vi "Parse Category Overrides.vi"() -> (1 "Non Localized Names":string[](array[string]), 2 "Names":string[](array[string]), 3 "Priorities":i32[](array[numeric]))   [LabVIEW 2016, in "NI_NPW_Filters.lvlib"]
uses:
  <resource>/dialog/NewProjectWizard/Filters/NI_NPW_Filters.lvlib
  <resource>/dialog/NewProjectWizard/Loading Project Info/NI_NPW_Loading Project Info.lvlib
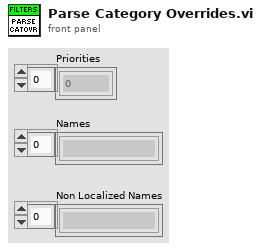
[diagram p1: front panel]
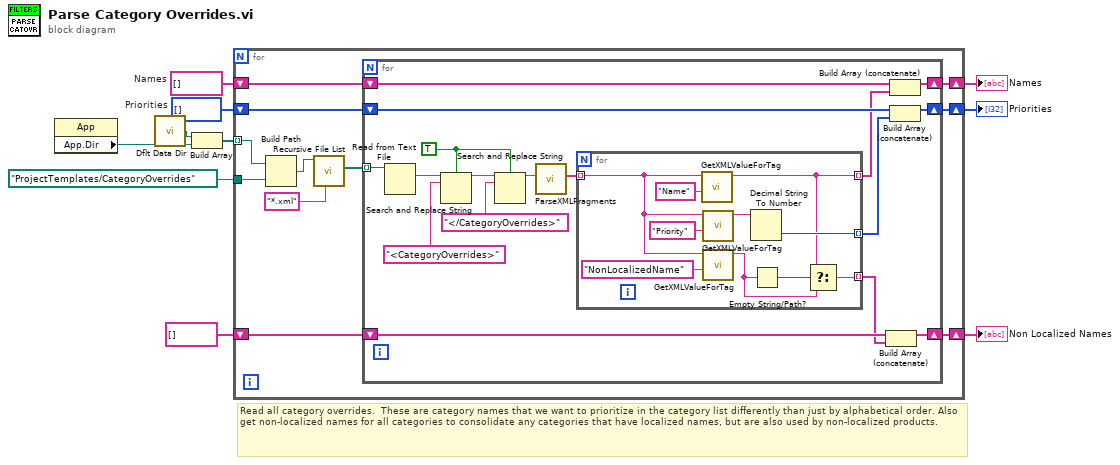
[diagram p0: block diagram]
diagram:
  w8 = i32[] []  # Priorities
  w7 = string[] []  # Names
  # "Read all category overrides.  These are category names that we want to prioritize in the category list differently than just by alphabetical order. Also get non-localized names for all categories to consolidate any categories that have localized names, but are also used by non-localized products."
  n1 = property class="App"() -> ("App.Dir"=w6:path)  [unwired: 2 in, 2 out]
  n2 = call <vilib>:"Dflt Data Dir.vi"() -> ("App:Default Data Directory"=w3:path)
  n3 = Build Array(w3, w6) -> (w4:path[])
  n4 = for {
    tunnel: w4 -> [w20] mode=indexing
    tunnel: path "ProjectTemplates/CategoryOverrides" -> [w21]
    shift-right: [w14] -> w9
    shift-left: w7 -> [w16]
    shift-right: [w13] -> w10
    shift-left: w8 -> [w15]
    shift-right: [w11] -> w1
    shift-left: string[] [] -> [w12]
    n5 = Build Path(base path=w20, name or relative path=w21) -> (appended path=w19:path)
    n6 = call <vilib>:"Recursive File List.vi"("pattern"="*.xml", "Folder Path"=w19) -> ("All Files in Dir"=w17:path[])  [unwired: 5 in, 4 out]
    n7 = for {
      tunnel: w17 -> [w38] mode=indexing
      shift-right: [w26] -> w14
      shift-left: w16 -> [w30]
      shift-right: [w25] -> w13
      shift-left: w15 -> [w29]
      shift-right: [w23] -> w11
      shift-left: w12 -> [w24]
      w34 = TRUE ("ignore case? (F)")
      n8 = Read from Text File(file (use dialog)=w38) -> (text=w36:string)  [unwired: 3 in, 3 out]
      n9 = Search and Replace String(case sensitive?=w34, input string=w36, search string="<CategoryOverrides>") -> (result string=w35:string)  [unwired: 5 in, 3 out]
      n10 = Search and Replace String(case sensitive?=w34, input string=w35, search string="</CategoryOverrides>") -> (result string=w32:string)  [unwired: 5 in, 3 out]
      n11 = call <vilib>:"ParseXMLFragments.vi"("XML in"=w32) -> ("XML Elements"=w37:string[])  [unwired: 9 in, 1 out]
      n12 = for {
        tunnel: w37 -> [w44] mode=indexing
        tunnel: [w40] -> w28 mode=indexing
        tunnel: [w45] -> w27 mode=indexing
        tunnel: [w39] -> w22 mode=indexing
        n13 = call <resource>:"GetXMLValueForTag.vi"("tag"="Name", "XML"=w44) -> ("value"=w40:string)  [unwired: 7 in, 2 out]
        n14 = call <resource>:"GetXMLValueForTag.vi"("tag"="Priority", "XML"=w44) -> ("value"=w46:string)  [unwired: 7 in, 2 out]
        n15 = call <resource>:"GetXMLValueForTag.vi"("tag"="NonLocalizedName", "XML"=w44) -> ("value"=w41:string)  [unwired: 7 in, 2 out]
        n16 = Decimal String To Number(string=w46) -> (number=w45:i32)  [unwired: 2 in, 1 out]
        n17 = Empty String/Path?(string/path=w41) -> (empty?=w42:bool)
        n18 = Select(t=w40, s=w42, f=w41) -> (s? t:f=w39:string)
      }
      n19 = Build Array (concatenate)(w24, w22) -> (w23:string[])
      n20 = Build Array (concatenate)(w30, w28) -> (w26:string[])
      n21 = Build Array (concatenate)(w29, w27) -> (w25:i32[])
    }
  }
  "Priorities" <- w10
  "Names" <- w9
  "Non Localized Names" <- w1
